vi "pixie gain shift.vi"(7 "shift control":string(combo)="read", 11 "gain":i32=1 min=1 max=200 step=1) -> (3 "gain out":i32)   [LabVIEW 2016]
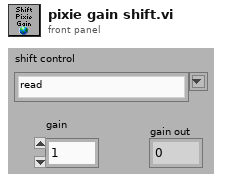
[diagram p1: front panel]
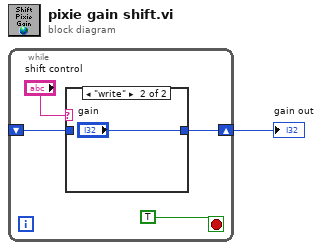
[diagram p0: block diagram]
diagram:
  n1 = while {
    shift-right: [w4] -> w1
    shift-left: _ -> [w2]
    stop <- TRUE ("stop") stop-if-true
    n2 = case shown="\"write\"" "shift control" {
      tunnel: [w6 "gain"] -> w4
      tunnel: w2 -> [w6 _]
      frame "read", Default {
      }
      frame "write" {
      }
    }
  }
  "gain out" <- w1
